vi "Save.vi"(8 "error in":errorcluster, 10 "file path":path, 11 "CEF_Hierachy repository in":refnum<class "CEF_HierarchyRepo.lvclass">) -> (0 "error out":errorcluster, 3 "CEF_Hierachy repository out":refnum<class "CEF_HierarchyRepo.lvclass">)   [LabVIEW 2025, in "CEF.lvlib" / "CEF_HierarchyRepo.lvclass"]
doc: "Stores repo information to file. It could save in multiple files or formats at the same time. File versioning is suggested.Copyright 2017 National Instruments Corporation\n\nLicensed under the Apache License, Version 2.0 (the \"License\"); you may not use this file except in compliance with the License. You may obtain a copy of the License at http://www.apache.org/licenses/LICENSE-2.0\nUnless required by applicable law or agreed to in writing, software distributed under the License is distributed on an \"AS IS\" BASIS, WITHOUT WARRANTIES OR CONDITIONS OF ANY KIND, either express or implied. See the License for the specific language governing permissions and limitations under the License."
uses:
  CEF_HierarchyRepo.lvclass
  CEF_HierarchyRepo.lvclass/CEF_HierarchyRepo.ctl
  CEF.lvlib
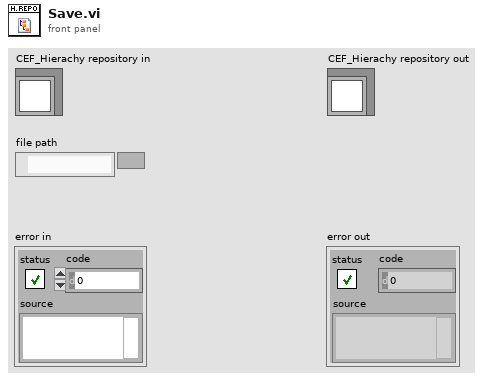
[diagram p1: front panel]
types:
  T1 = typedef "CEF.lvlib/CEF_HierarchyRepo.lvclass/memory hierarchy.ctl" = cluster{"hierarchy structure":T2, "instance data":refnum<class "CEF_serializable configuration.lvclass">[]}
  T2 = typedef "CEF.lvlib/CEF_HierarchyRepo.lvclass/full hierarchy.ctl" = cluster{"root":string, "hierarchy":T3[]}
  T3 = typedef "CEF.lvlib/hierarchy element.ctl" = cluster{"current node":string, "children":string[]}
  T4 = typedef "CEF.lvlib/flat hierarchy.ctl" = cluster{"hierarchy structure":T2, "instance data":T5[]}
  T5 = typedef "CEF.lvlib/instance data.ctl" = cluster{"ID":string, "Alias":string, "class":string, "version":string, "data":string}
  T6 = typedef "CEF.lvlib/base file format.ctl" = cluster{"version":string, "data":string}
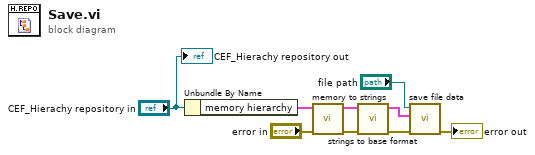
[diagram p0: block diagram]
diagram:
  n1 = Unbundle By Name("CEF_Hierachy repository in") -> ("memory hierarchy"=w4:T1)
  n2 = call "memory to strings.vi"("error in"="error in", "memory hierarchy"=w4) -> ("error out"=w3:errorcluster, "1.0.0"=w1:T4)  [unwired: 8 in]
  n3 = call "strings to base format.vi"("error in"=w3, "1.0.0"=w1) -> ("error out"=w6:errorcluster, "format"=w5:T6)  [unwired: 8 in]
  n4 = call "save file data.vi"("error in"=w6, "format"=w5, "Path"="file path") -> ("error out"=→"error out":errorcluster)  [unwired: 8 in]
  "CEF_Hierachy repository out" <- "CEF_Hierachy repository in"
